vi "PH_Sequencer.PC SetPPMAGUIElements.vi"(0 "i ref in":refnum<vi>, 5 "error in (no error)":errorcluster) -> (14 "i ref out":refnum<vi>, 19 "error out":errorcluster)   [LabVIEW 2014, in "PH_Sequencer.lvlib"]
doc: "This VI enables or disables the GUI elements depending on the MainAmp-Freigabe."
uses:
  PH_Sequencer.lvlib
  PH_Basics/PH_PP_Common/PH_PP_Common.PUs.ctl
  PH_Basics/PH_StatusHandler/PH_StatusHandler.Status.ctl
  PH_Basics/PH_SystemInformation/PH_SystemInformation.lvlib
  PH_BeamlineInformation/PH_BeamlineInformation.lvlib
  PH_Basics/PH_PP_Common/PH_PP_Common.lvlib
  PH_Basics/PH_StatusHandler/PH_StatusHandler.lvlib
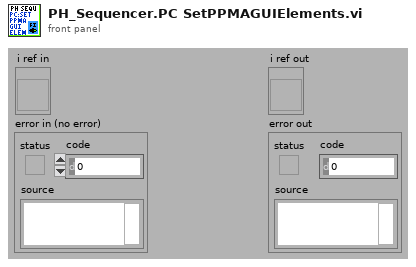
[diagram p1: front panel]
types:
  T1 = typedef "PH_StatusHandler.lvlib/PH_StatusHandler.Status.ctl" = i16
  T2 = typedef "PH_PP_Common.lvlib/PH_PP_Common.PUs.ctl" = enum16{"no Info", "PA-19mm-1", "PA-19mm-2", "PA-45mm-PILC", "PA-45mm-MAIN", "MA-PU-1", "MA-PU-2", "MA-PU-3", "MA-PU-4", "MA-PU-5", "MA-PU-6", "MA-FR", "MA-PILC", "PA-45mm-DP"}
  T3 = enum16{"Laser", "PreAmp", "MainAmp", "Exp 1", "Exp 2", "Exp 3", "Exp 4"}
  T4 = typedef "PH_Sequencer.lvlib/PH_Sequencer.i attribute.ctl" = cluster{"GUI Refs":cluster{"Main Off":refnum<vi>, "Fire":refnum<vi>, "Status":refnum<vi>, "Ready":refnum<vi>, "Waiting Time":refnum<vi>, "Timeout":refnum<vi>, "PPMA Ready":refnum<vi>, "Sequencer SM State":refnum<vi>, "PPPA Ready":refnum<vi>, "Calorimeter":refnum<vi>, "Beamline Ready":refnum<vi>, "Clear Beamline":refnum<vi>, "Linkage PPMA Rods":refnum<vi>, "Linkage Current PA":refnum<vi>, "Linkage Current MA":refnum<vi>, "Timing Ready":refnum<vi>, "State Timing":refnum<vi>, "Force Timing":refnum<vi>, "PSDB Shot Comment":refnum<vi>, "State PA Backreflection":refnum<vi>, "Beamline Z6 Ready":refnum<vi>, "Clear Z6 Beamline":refnum<vi>, "Sequence length":refnum<vi>, "Timing Mode":refnum<vi>, "Slow Trigger Settings":refnum<vi>, "Experiment Description":refnum<vi>, "State PSDB":refnum<vi>, "PSDB Ready":refnum<vi>, "Set PSDB Settings":refnum<vi>, "Get PSDB Info":refnum<vi>, "Take Snapshot":refnum<vi>, "Shottype":refnum<vi>, "Experiment":refnum<vi>, "Phase Frontends":refnum<vi>, "PP 45mm PILC in use":refnum<vi>}, "Status Info":cluster{"Machine Status":T1, "WaitingTime":i32, "Timeout":bool}, "Readyness":cluster{"Ready to shot":bool, "PPMA Ready":bool, "PPPA Ready":bool, "BL Ready":bool, "Timing Ready":bool, "BL Z6 Ready":bool, "PSDBReady":bool}, "Instancenames":cluster{"PPMA Rods":string, "PP Current Meas":string, "PH Beamline Chief":string, "PA Backrefl Meas":string, "Z6 Beamline Chief":string}, "Data to read":bool, "Calorimeter":cluster{"Instancename":string, "On":bool, "linked":bool}, "Linkage":cluster{"PPMA Rods":bool, "PP Current Meas":bool, "PHELIX Beamline Chief":bool, "PA Backrefl Meas":bool, "Z6 Beamline Chief":bool}, "Timing":cluster{"Instance":string, "linked":bool, "Status":T1, "Timing Mode":T5, "Slow Trigger Settings":T6, "Info available":cluster{"ext SlowTrigger":bool, "T2":bool, "Mode":bool, "Delay Slow Trigger":bool, "Phase FEs":bool}, "FE Phase":T7}, "Service ID R2S":i32, "PSDB":cluster{"Controller Instance":string, "Controller Status":T1, "Controller linked":bool, "Settings acknowledged":bool, "Current Experiment ID":i16, "Current Shot Type":i16, "Current Comment":string, "Remember Settings":bool, "Write 2 early":bool}, "PSDB Data":cluster{"Main Off?":bool, "Sequence Length":dbl, "Sequence startet":timestamp}, "6P 4Q Positions":cluster{"Instancename":string, "linked":bool, "Position":T8}[], "PUs":T9[]}
  T5 = typedef "PH_Timing.lvlib/PH_Timing.Timing Mode.ctl" = cluster{"T2":i16, "Modeselector":enum32{"10 Hz", "0.5 Hz", "Shot"}}
  T6 = typedef "PH_Timing.lvlib/PH_Timing.Slow Trigger Settings.ctl" = cluster{"Delay":dbl, "externally triggered?":bool}
  T7 = typedef "PH_Timing.lvlib/PH_Timing.Phase FEs.ctl" = cluster{"Phase":dbl}
  T8 = typedef "PH_4_Pos_Selector.lvlib/PH_4_Pos_Selector.Position Selector.ctl" = u16
  T9 = typedef "PH_Sequencer.lvlib/PH_Sequencer.Head.ctl" = cluster{"PowerUnit":T2, "GUI Ref":refnum<vi>, "Information":T10, "linked?":bool, "GUI Ref Current Voltage":refnum<vi>}
  T10 = typedef "PH_Sequencer.lvlib/PH_Sequencer.PU Information.ctl" = cluster{"State":T1, "Waiting Time [s]":dbl, "PU State SM":T11, "PU Timeout SM":T11}
  T11 = typedef "PH_PowerUnit_BaseClass.lvlib/PH_PowerUnit_BaseClass.SM States.ctl" = enum16{".", "Stand by", "Switch PU on", "Configure", "Set Default Voltage", "Set STANDBY", "Set READY", "Wait for Shot Cmd", "Open Dump Rods", "Open Ross Relais", "Close Ross Relais", "Switch PSU on", "Switch PSU off", "Charge", "Switch GD Channel on", "Close Dump Rods", "Rods-TO", "RR-TO", "PSU-TO", "Trigger-TO"}
  T12 = typedef "PH_SystemInformation.lvlib/PH_SystemInformationEnabling State.ctl" = i32
  T13 = typedef "PH_BeamlineInformation.lvlib/PH_BeamlineInformation.i attribute.ctl" = cluster{"BL GUI Elements of Services":cluster{"Service Name":string, "GUI Elements":refnum<vi>[], "Status":i32}[], "Powermeters":T14, "Efficiency":T15, "Heads":T16[]}
  T14 = typedef "PH_BeamlineInformation.lvlib/PH_BeamlineInformation.Powermeter.ctl" = cluster{"ns FE":cluster{"GUI Ref":refnum<vi>, "Value":dbl}, "fs FE":cluster{"GUI Ref":refnum<vi>, "Value":dbl}, "PA":cluster{"GUI Ref":refnum<vi>, "Value":dbl}, "MA":cluster{"GUI Ref":refnum<vi>, "Value":dbl}, "Z6 green":cluster{"GUI Ref":refnum<vi>, "Value":dbl}, "Z6 IR":cluster{"GUI Ref":refnum<vi>, "Value":dbl}, "Z6 COS":cluster{"GUI Ref":refnum<vi>, "Value":dbl}}
  T15 = typedef "PH_BeamlineInformation.lvlib/PH_BeamlineInformation.Efficiency.ctl" = cluster{"PA Gain":cluster{"GUI Ref":refnum<vi>, "Value":dbl}, "MA Gain":cluster{"GUI Ref":refnum<vi>, "Value":dbl}, "Z6 green Conversion":cluster{"GUI Ref":refnum<vi>, "Value":dbl}, "Z6 Comp Losses":cluster{"GUI Ref":refnum<vi>, "Value":dbl}}
  T16 = typedef "PH_BeamlineInformation.lvlib/PH_BeamlineInformation.Head.ctl" = cluster{"PowerUnit":T2, "in use":cluster{"Value":bool, "GUI Ref":refnum<vi>, "linked":bool}, "voltage":cluster{"Value":dbl, "GUI Ref":refnum<vi>, "linked":bool}}
  T17 = enum8{"Enabled", "Disabled", "Disabled and Grayed Out"}
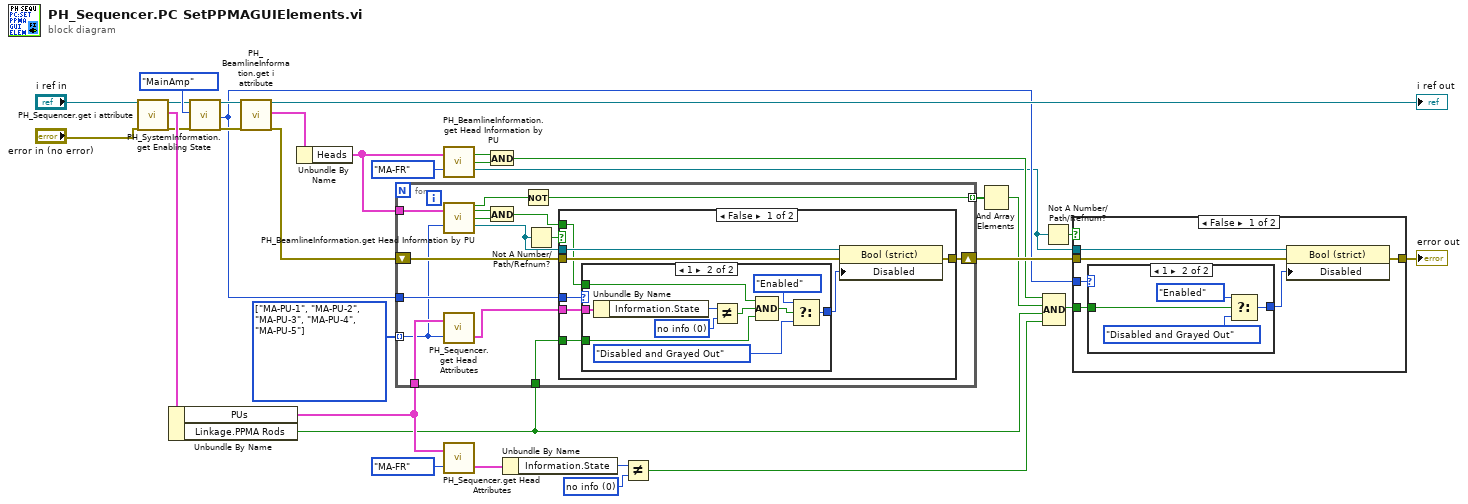
[diagram p0: block diagram]
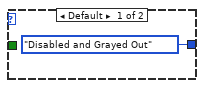
[diagram p2: hidden frame]
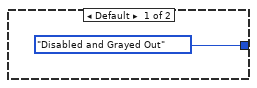
[diagram p4: hidden frame]
diagram:
  w2 = T1 0 items=["no info", "off/false/out", "on/true/in", "Failure", "Alarm", "Status 1", "Status 2", "Status 3"] ("y")
  w13 = T2[] [enum."MA-PU-1", enum."MA-PU-2", enum."MA-PU-3", enum."MA-PU-4", enum."MA-PU-5"] items=["no Info", "PA-19mm-1", "PA-19mm-2", "PA-45mm-PILC", "PA-45mm-MAIN", "MA-PU-1", "MA-PU-2", "MA-PU-3", "MA-PU-4", "MA-PU-5", "MA-PU-6", "MA-FR", "MA-PILC", "PA-45mm-DP"]
  n1 = call "PH_Sequencer.get i attribute.vi"("i ref in"="i ref in", "error in (no error)"="error in (no error)") -> ("i ref out"=w27:refnum<vi>, "i attribute"=w32:T4, "error out"=w26:errorcluster)  [unwired: 15 in]
  n2 = Unbundle By Name(w32) -> ("PUs"=w6:T9[], "Linkage.PPMA Rods"=w1:bool)
  n3 = call "PH_SystemInformation.get Enabling State.vi"("i ref in"=w27, "Wanted State"=T3."MainAmp", "error in (no error)"=w26) -> ("i ref out"=w25:refnum<vi>, "Enabling State"=w16:T12, "error out"=w24:errorcluster)  [unwired: 14 in]
  n4 = call "PH_BeamlineInformation.get i attribute.vi"("i ref in"=w25, "error in (no error)"=w24) -> ("i ref out"=→"i ref out":refnum<vi>, "i attribute"=w28:T13, "error out"=w22:errorcluster)  [unwired: 15 in]
  n5 = Unbundle By Name(w28) -> ("Heads"=w10:T16[])
  n6 = for {
    shift-right: [w46] -> w21
    shift-left: w22 -> [w47]
    tunnel: w16 -> [w45]
    tunnel: w1 -> [w44]
    tunnel: w6 -> [w41]
    tunnel: w13 -> [w36] mode=indexing
    tunnel: w10 -> [w35]
    tunnel: [w33] -> w5 mode=indexing
    n7 = call "PH_BeamlineInformation.get Head Information by PU.vi"("Heads"=w35, "Power Unit"=w36) -> ("In Use?"=w34:bool, "In Use linked?"=w39:bool, "Voltage linked?"=w38:bool, "In Use GUI Ref"=w37:refnum<vi>)  [unwired: 12 in, 2 out]
    n8 = call "PH_Sequencer.get Head Attributes.vi"("PowerUnit"=w36, "Heads"=w41) -> ("Head"=w40:T9)  [unwired: 1 out]
    n9 = And(x=w39, y=w38) -> (x .and. y?=w42:bool)
    n10 = Not(x=w34) -> (.not. x?=w33:bool)
    n11 = Not A Number/Path/Refnum?(number/path/refnum=w37) -> (NaN/Path/Refnum?=w43:bool)
    n12 = case shown="False" w43 {
      tunnel: w37 -> [w55 _]
      tunnel: w47 -> [w54 w67]
      tunnel: [w53 w67] -> w46
      tunnel: w45 -> [w52 _]
      tunnel: w44 -> [w51 _]
      tunnel: w40 -> [w49 _]
      tunnel: w42 -> [w48 _]
      frame False {
        n13 = case shown="1" w52 {
          tunnel: [T17."Disabled and Grayed Out" ("Disabled") w64] -> w50
          tunnel: w51 -> [_ w66]
          tunnel: w49 -> [_ w61]
          tunnel: w48 -> [_ w60]
          frame Default {
          }
          frame 1 {
            w57 = T1 0 items=["no info", "off/false/out", "on/true/in", "Failure", "Alarm", "Status 1", "Status 2", "Status 3"] ("y")
            n14 = Unbundle By Name(w61) -> ("Information.State"=w59:T1)
            n15 = Not Equal?(x=w59, y=w57) -> (x != y?=w58:bool)
            n16 = Compound Arithmetic op=AND(w60, w58, w66) -> (w65:bool)
            n17 = Select(t=T17."Enabled", s=w65, f=T17."Disabled and Grayed Out" ("Disabled")) -> (s? t:f=w64:T17)
          }
        }
        n18 = property class="Bool (strict)"(reference=w55, error in=w54, "Disabled"=w50) -> (error out=w53:errorcluster)  [unwired: 1 out]
      }
      frame True {
      }
    }
  }
  n19 = call "PH_BeamlineInformation.get Head Information by PU.vi"("Heads"=w10, "Power Unit"=PH_PP_Common.PUs."MA-FR") -> ("In Use linked?"=w9:bool, "Voltage linked?"=w8:bool, "In Use GUI Ref"=w11:refnum<vi>)  [unwired: 12 in, 3 out]
  n20 = call "PH_Sequencer.get Head Attributes.vi"("PowerUnit"=PH_PP_Common.PUs."MA-FR", "Heads"=w6) -> ("Head"=w14:T9)  [unwired: 1 out]
  n21 = And(x=w9, y=w8) -> (x .and. y?=w12:bool)
  n22 = Unbundle By Name(w14) -> ("Information.State"=w4:T1)
  n23 = Not Equal?(x=w4, y=w2) -> (x != y?=w3:bool)
  n24 = And Array Elements(Boolean array=w5) -> (logical AND=w18:bool)
  n25 = Not A Number/Path/Refnum?(number/path/refnum=w11) -> (NaN/Path/Refnum?=w19:bool)
  n26 = Compound Arithmetic op=AND(w12, w18, w1, w3) -> (w17:bool)
  n27 = case shown="False" w19 {
    tunnel: w21 -> [w73 w79]
    tunnel: [w72 w79] -> w20
    tunnel: w11 -> [w71 _]
    tunnel: w17 -> [w70 _]
    tunnel: w16 -> [w69 _]
    frame False {
      n28 = case shown="1" w69 {
        tunnel: [T17."Disabled and Grayed Out" ("Disabled") w78] -> w68
        tunnel: w70 -> [_ w75]
        frame Default {
        }
        frame 1 {
          n29 = Select(t=T17."Enabled", s=w75, f=T17."Disabled and Grayed Out" ("Disabled")) -> (s? t:f=w78:T17)
        }
      }
      n30 = property class="Bool (strict)"(reference=w71, error in=w73, "Disabled"=w68) -> (error out=w72:errorcluster)  [unwired: 1 out]
    }
    frame True {
    }
  }
  "error out" <- w20
